vi "CamDef.vi"() -> ()   [LabVIEW 2011]
panel:
  out "CamDef":bool
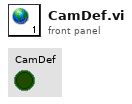
[diagram p1: front panel]
diagram:
